vi "Do.vi"(8 "error in (no error)":errorcluster, 10 "Actor in":refnum<class "Actor.lvclass">, 11 "Data Tracker Msg":refnum<class "Data Tracker Msg.lvclass">) -> (0 "error out":errorcluster, 2 "Actor out":refnum<class "Actor.lvclass">)   [LabVIEW 2020, in "Data Tracker.lvlib" / "Data Tracker Msg.lvclass"]
doc: "This Do implementation will forward itselft to the Data Tracker. On the Data Tracker actor it will call the parent method."
uses:
  Data Tracker Msg.lvclass
  C:/Current projects/WS/PPL/HDH.Actor Framework.Core.Publisher.lvlibp/Messages/Response Msg/Response Msg.lvclass
  PPL/HDH.Actor Framework.Core.Actor.lvlibp/1abvi3w/vi.lib/ActorFramework/Actor/Actor.lvclass
  Data Tracker/Data Tracker.lvclass
  C:/Current projects/WS/PPL/HDH.Actor Framework.Core.Actor.lvlibp/1abvi3w/vi.lib/ActorFramework/Actor/Actor.lvclass
  Data Tracker Msg.lvclass/Data Tracker Msg.ctl
  PPL/HDH.Actor Framework.Core.Publisher.lvlibp/Publisher Messages/Targetted Msg/Targetted Msg.lvclass
  C:/Current projects/WS/PPL/HDH.Actor Framework.Core.Publisher.lvlibp/Publisher Messages/Sender Msg/Sender Msg.lvclass
  PPL/HDH.Actor Framework.Core.Publisher.lvlibp/Messages/Timed Msg/Timed Msg.lvclass
  PPL/HDH.Actor Framework.Core.Publisher.lvlibp/Messages/Response Msg/Response Msg.lvclass
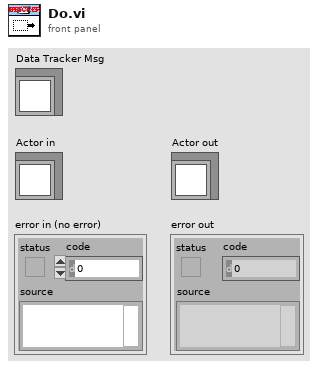
[diagram p1: front panel]
types:
  T1 = typedef "HDH.Actor Framework.Core.Actor.lvlibp/Message Enqueuer.lvclass/Message Priority.ctl" = enum16{"Low", "Normal", "High"}
  T2 = typedef "HDH.Actor Framework.Core.Publisher.lvlibp/Ctl_SendFunction.ctl" = enum16{"Send and Forget", "Request Reply", "Await Reply"}
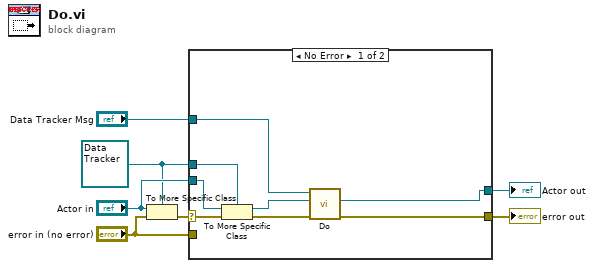
[diagram p0: block diagram]
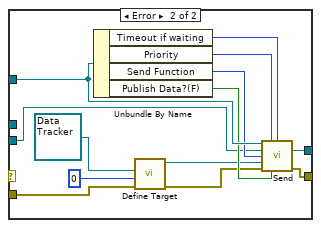
[diagram p2: hidden frame]
diagram:
  w1 = refnum<class "Data Tracker.lvclass"> refnum ("Data Tracker.lvlib:Data Tracker.lvclass")
  n1 = To More Specific Class(target class=w1, reference="Actor in", error in="error in (no error)") -> (error out=w4:errorcluster)  [unwired: 1 out]
  n2 = case shown="No Error" w4 {
    selector: w4 -> [w12 _]
    tunnel: [w15 w16] -> w7
    tunnel: [w14 w17] -> w6
    tunnel: "Data Tracker Msg" -> [w13 w28]
    tunnel: "error in (no error)" -> [_ w21]
    tunnel: "Actor in" -> [w10 w19]
    tunnel: w1 -> [w9 _]
    frame No Error {
      n3 = To More Specific Class(target class=w9, reference=w10, error in=w12) -> (specific class reference=w8:refnum<class "Data Tracker.lvclass">, error out=w11:errorcluster)
      n4 = call-parent "Do.vi"("error in (no error)"=w11, "Actor in"=w8, "Response Msg"=w13) -> ("error out"=w15:errorcluster, "Actor out"=w14:refnum<class "Actor.lvclass">)  [unwired: 7 in]
    }
    frame Error {
      n5 = Unbundle By Name(w28) -> ("Timeout if waiting"=w26:i32, "Priority"=w27:T1, "Send Function"=w25:T2, "Publish Data?(F)"=w24:bool)
      n6 = call "Define Target.vi"("error in (no error)"=w21, "Target Actor index(-1, all)"=0, "Target Actor"=refnum<class "Data Tracker.lvclass"> refnum ("Data Tracker.lvlib:Data Tracker.lvclass")) -> ("error out"=w18:errorcluster, "Targetted Msg out"=w20:refnum<class "Targetted Msg.lvclass">)  [unwired: 7 in]
      n7 = call "Send.vi"("Response Msg in"=w28, "Message Priority (Normal)"=w27, "Timeout if waiting(-1ms)"=w26, "Actor in"=w19, "Send Function"=w25, "Sender (publish)"=w20, "error in (no error)"=w18, "Publish Data?(F)"=w24) -> ("Actor out"=w17:refnum<class "Actor.lvclass">, "error out"=w16:errorcluster)  [unwired: 3 in, 3 out]
    }
  }
  "error out" <- w7
  "Actor out" <- w6
